vi "Movie_grabframe.vi"(8 "error in (no error)":errorcluster, 9 "path to PNG file":path, 10 "frame number":i32=12, 11 "Path":path) -> (0 "error out":errorcluster, 1 "return value":u8[][][](array[numeric]), 2 "attributes":T2, 3 "new picture":picture, 4 "image data":T1)   [LabVIEW 2025]
uses:
  <vilib>/picture/picture.llb/Draw True-Color Pixmap.vi
  <vilib>/picture/picture.llb/imagedata.ctl
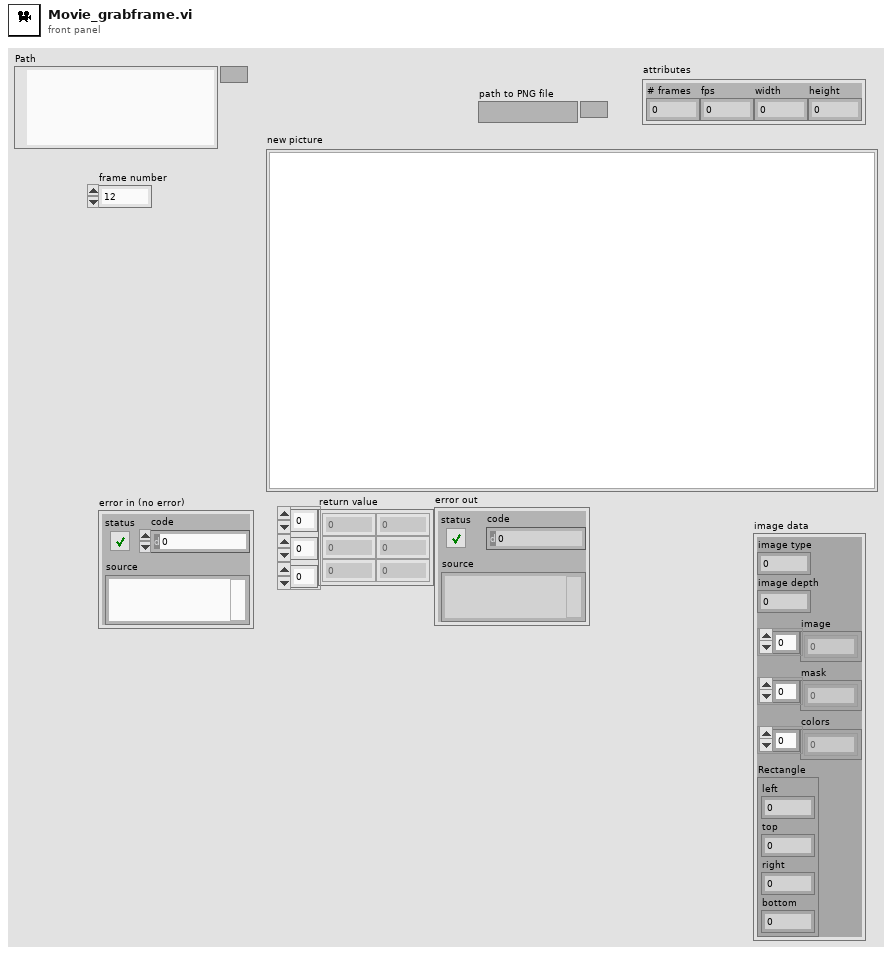
[diagram p1: front panel]
types:
  T1 = typedef "imagedata.ctl" = cluster{"image type":i32, "image depth":i32, "image":u8[], "mask":u8[], "colors":u32[], "Rectangle":cluster{"left":i16, "top":i16, "right":i16, "bottom":i16}}
  T2 = cluster{"# frames":i32, "fps":i32, "width":i32, "height":i32}
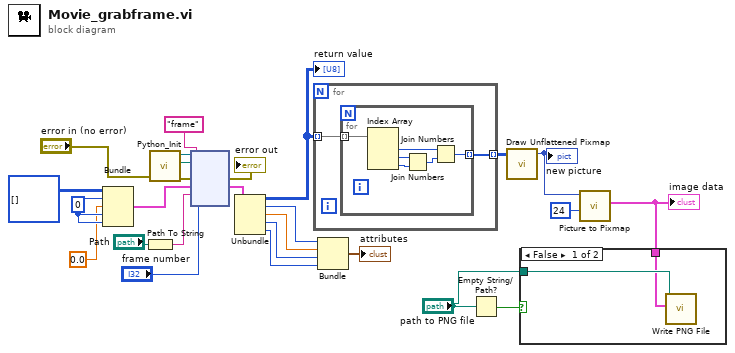
[diagram p0: block diagram]
diagram:
  w12 = 0
  n1 = Bundle(u8[][][] [], w12, 0.0, w12, w12) -> (w13:cluster{u8[][][], i32, dbl, i32, i32})  [unwired: 1 in]
  n2 = Path To String(path="Path") -> (string=w18:string)
  n3 = call "Python_Init.vi"("error in (no error)"="error in (no error)") -> ("Refnum out"=w21:refnum<k35>, "code"=w22:path, "error out"=w23:errorcluster)  [unwired: 3 in]
  n4 = node ("Python Node")(w21, w22, "frame" ("function name"), w23, w13, w18, "frame number") -> (→"error out":errorcluster, w17:cluster{u8[][][], i32, dbl, i32, i32})  [unwired: 2 in, 3 out]
  n5 = Unbundle(w17) -> (w14:u8[][][], w10:i32, w9:dbl, w8:i32, w7:i32)
  "return value" <- w14
  n6 = for {
    tunnel: w14 -> [w28] mode=indexing
    tunnel: [w27] -> w26 mode=indexing
    n7 = for {
      tunnel: w28 -> [w34] mode=indexing
      tunnel: [w29] -> w27 mode=indexing
      n8 = Index Array(array=w34) -> (element #1=w31:u8, element #2=w32:u8, element #3=w33:u8)  [unwired: 3 in]
      n9 = Join Numbers(hi=w32, lo=w33) -> ((hi.lo)=w30:u16)
      n10 = Join Numbers(hi=w31, lo=w30) -> ((hi.lo)=w29:u32)
    }
  }
  n11 = Bundle(w10, w9, w8, w7) -> (→"attributes":cluster{i32, dbl, i32, i32})  [unwired: 1 in]
  n12 = Empty String/Path?(string/path="path to PNG file") -> (empty?=w4:bool)
  n13 = call-poly <vilib>:"Draw Unflattened Pixmap.vi"("data (RGB format)"=w26) -> ("new picture"=w5:picture)  [unwired: 8 in]
  "new picture" <- w5
  n14 = call <vilib>:"Picture to Pixmap.vi"("depth"=24, "picture"=w5) -> ("image data"=w1:T1)  [unwired: 8 in, 1 out]
  "image data" <- w1
  n15 = case shown="False" w4 {
    tunnel: "path to PNG file" -> [w36 _]
    tunnel: w1 -> [w35 _]
    frame False {
      n16 = call <vilib>:"Write PNG File.vi"("image data"=w35, "path to PNG file"=w36) -> ()  [unwired: 8 in, 2 out]
    }
    frame True {
    }
  }
